vi "S2C_VLFT10_Proc_RfPathSelect.vi"(8 "Error In":errorcluster, 9 "DiffProbe?":bool, 10 "Active?":bool, 11 "HandSwitch":T1 items=["Mono1 Cut", "Mono1 Coag", "Mono2 Cut", "Mono2 Coag", "Mono2 ValleyLab", "Bipolar", "LXF Bipolar", "Ligasure", "LXF Ligasure"]) -> (0 "Error Out":errorcluster, 3 "Result":string)   [LabVIEW 2015]
uses:
  Typedefs/S2C_VLFT10_Type_HandSwitch.ctl
  PCIe7841/VIs/Typedefs/S2C_PCIe7841_Type_PathRelayWr.ctl
  PCIe7841/VIs/Typedefs/S2C_PCIe7841_Type_PathRelayRd.ctl
  PCIe7841/VIs/Typedefs/S2C_PCIe7841_Type_RemWr.ctl
  PCIe7841/VIs/Typedefs/S2C_PCIe7841_Type_RemRd.ctl
  PCIe7841/VIs/PolyDriver/S2C_PCIe7841_Poly_RelayPathWrite.vi
  PCIe7841/VIs/PolyDriver/S2C_PCIe7841_Poly_RelayPathRead.vi
  PCIe7841/VIs/PolyDriver/S2C_PCIe7841_Poly_RemWrite.vi
  PCIe7841/VIs/PolyDriver/S2C_PCIe7841_Poly_RemRead.vi
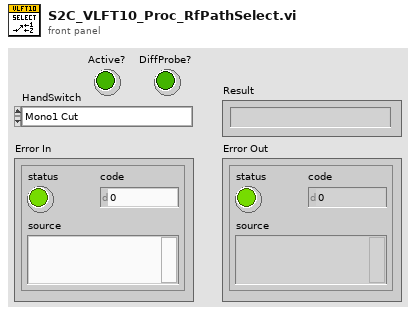
[diagram p1: front panel]
types:
  T1 = typedef "S2C_VLFT10_Type_HandSwitch.ctl" = u16
  T2 = typedef "S2C_PCIe7841_Type_RemRd.ctl" = string
  T3 = typedef "S2C_PCIe7841_Type_RemWr.ctl" = string
  T4 = typedef "S2C_PCIe7841_Type_PathRelayRd.ctl" = string
  T5 = typedef "S2C_PCIe7841_Type_PathRelayWr.ctl" = string
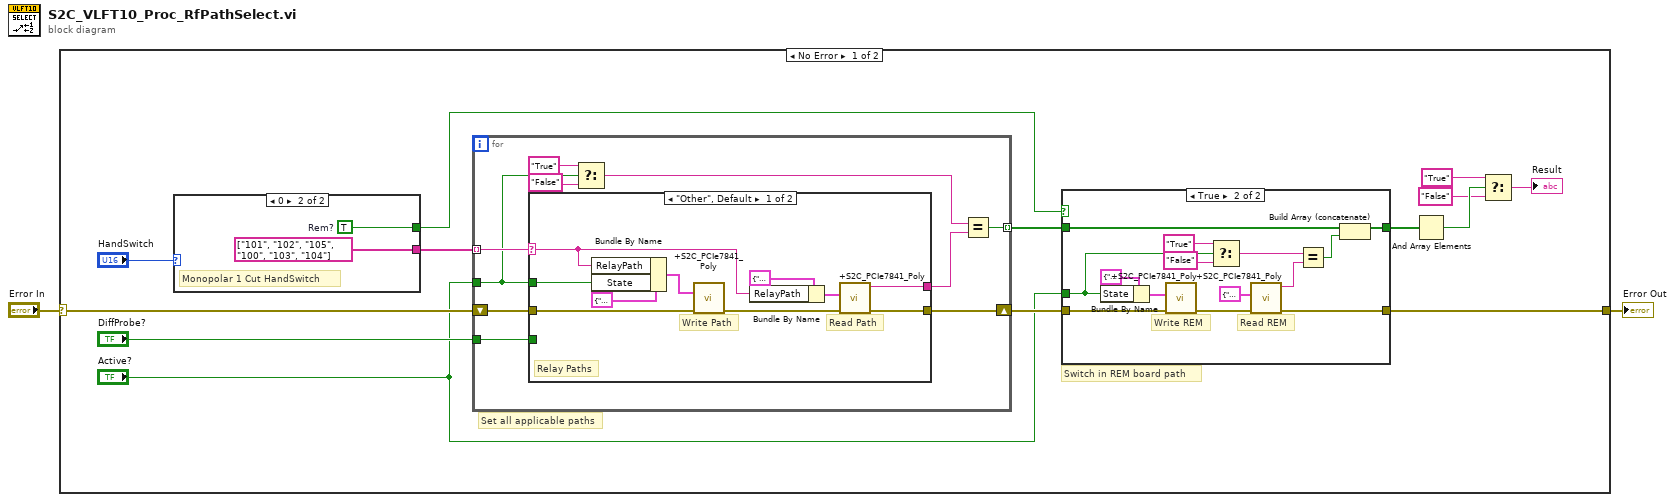
[diagram p0: block diagram]
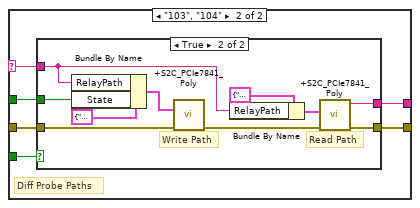
[diagram p3: hidden frame]
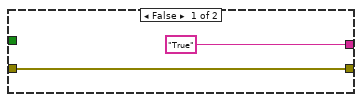
[diagram p4: hidden frame]
diagram:
  n1 = case shown="No Error" "Error In" {
    selector: "Error In" -> [w5 w73]
    tunnel: [w3 w73] -> w2
    frame No Error {
      # "Set all applicable paths"
      # "Switch in REM board path"
      n2 = case shown="0" "HandSwitch" {
        tunnel: [_ T5[] ["101", "102", "105", "100", "103", "104"]] -> w11
        tunnel: [_ w71] -> w8
        frame 99, Default {
        }
        frame 0 {
          w71 = TRUE  # Rem?
          # "Monopolar 1 Cut HandSwitch"
        }
      }
      n3 = for {
        shift-right: [w41] -> w10
        shift-left: w5 -> [w40]
        tunnel: [w42] -> w7 mode=indexing
        tunnel: "DiffProbe?" -> [w39]
        tunnel: w11 -> [w38] mode=indexing
        tunnel: "Active?" -> [w35]
        n4 = case shown="\"Other\", Default" w38 {
          selector: w38 -> [w49 w55]
          tunnel: [w52 w58] -> w41
          tunnel: w40 -> [w51 w57]
          tunnel: [w50 w56] -> w33
          tunnel: w39 -> [_ w54]
          tunnel: w35 -> [w48 w53]
          frame "Other", Default {
            # "Read Path"
            # "Write Path"
            # "Relay Paths"
            n5 = Bundle By Name(cluster=cluster{"RelayPath":T5, "State":bool} {"RelayPath"="110", "State"=TRUE} ("RelayPath"), "RelayPath"=w49, "State"=w48) -> (w47:cluster{"RelayPath":T5, "State":bool})
            n6 = call-poly "+S2C_PCIe7841_Poly.vi"("Error In"=w51, "RelayPath"=w47) -> ("Error Out"=w45:errorcluster)  [unwired: 8 in, 1 out]
            n7 = Bundle By Name(cluster=cluster{"RelayPath":T4} {"RelayPath"="110"} ("RelayPath"), "RelayPath"=w49) -> (w43:cluster{"RelayPath":T4})
            n8 = call-poly "+S2C_PCIe7841_Poly.vi"("Error In"=w45, "RelayPath"=w43) -> ("Error Out"=w52:errorcluster, "Response"=w50:string)  [unwired: 8 in]
          }
          frame "103", "104" {
            # "Diff Probe Paths"
            n9 = case shown="True" w54 {
              tunnel: [w60 w62] -> w58
              tunnel: w57 -> [w60 w69]
              tunnel: ["True" ("Response") w61] -> w56
              tunnel: w55 -> [_ w64]
              tunnel: w53 -> [_ w67]
              frame False {
              }
              frame True {
                # "Read Path"
                # "Write Path"
                n10 = Bundle By Name(cluster=cluster{"RelayPath":T5, "State":bool} {"RelayPath"="110", "State"=TRUE} ("RelayPath"), "RelayPath"=w64, "State"=w67) -> (w70:cluster{"RelayPath":T5, "State":bool})
                n11 = call-poly "+S2C_PCIe7841_Poly.vi"("Error In"=w69, "RelayPath"=w70) -> ("Error Out"=w66:errorcluster)  [unwired: 8 in, 1 out]
                n12 = Bundle By Name(cluster=cluster{"RelayPath":T4} {"RelayPath"="110"} ("RelayPath"), "RelayPath"=w64) -> (w63:cluster{"RelayPath":T4})
                n13 = call-poly "+S2C_PCIe7841_Poly.vi"("Error In"=w66, "RelayPath"=w63) -> ("Error Out"=w62:errorcluster, "Response"=w61:string)  [unwired: 8 in]
              }
            }
          }
        }
        n14 = Select(t="True", s=w35, f="False") -> (s? t:f=w34:string)
        n15 = Equal?(x=w34, y=w33) -> (x = y?=w42:bool)
      }
      n16 = case shown="True" w8 {
        tunnel: w10 -> [w17 w32]
        tunnel: w7 -> [w18 w31]
        tunnel: [w17 w25] -> w3
        tunnel: [w18 w30] -> w6
        tunnel: "Active?" -> [_ w22]
        frame False {
          # "Rem not required"
        }
        frame True {
          # "Read REM"
          # "Write REM"
          n17 = Bundle By Name(cluster=cluster{"REM":T3, "State":bool} {"REM"="121", "State"=FALSE} ("REM"), "State"=w22) -> (w28:cluster{"REM":T3, "State":bool})
          n18 = call-poly "+S2C_PCIe7841_Poly.vi"("Error In"=w32, "REM"=w28) -> ("Error Out"=w27:errorcluster)  [unwired: 8 in, 1 out]
          n19 = Select(t="True", s=w22, f="False") -> (s? t:f=w20:string)
          n20 = call-poly "+S2C_PCIe7841_Poly.vi"("Error In"=w27, "REM"=cluster{"REM":T2} {"REM"="121"}) -> ("Error Out"=w25:errorcluster, "Response"=w21:string)  [unwired: 8 in]
          n21 = Equal?(x=w20, y=w21) -> (x = y?=w19:bool)
          n22 = Build Array (concatenate)(w31, w19) -> (w30:bool[])
        }
      }
      n23 = And Array Elements(Boolean array=w6) -> (logical AND=w15:bool)
      n24 = Select(t="True", s=w15, f="False") -> (s? t:f=→"Result":string)
    }
    frame Error {
    }
  }
  "Error Out" <- w2
